vi "LVClass_HasoData Read HasoData - property.vi"(8 "error in (no error)":errorcluster, 11 "HasoData in":refnum<class "HasoData.lvclass">) -> (0 "error out":errorcluster, 2 "HasoData":T1, 3 "HasoData out":refnum<class "HasoData.lvclass">)   [LabVIEW 2020, in "HasoData.lvclass"]
uses:
  HasoData.lvclass
  Controls/ClassID.ctl
  HasoData.lvclass/HasoData.ctl
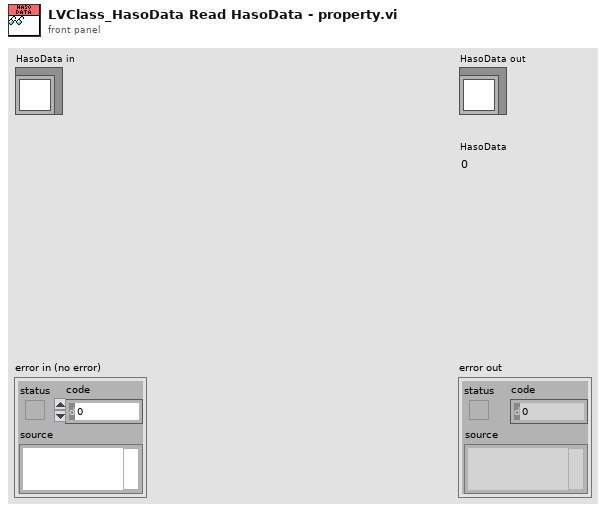
[diagram p1: front panel]
types:
  T1 = typedef "ClassID.ctl" = i64
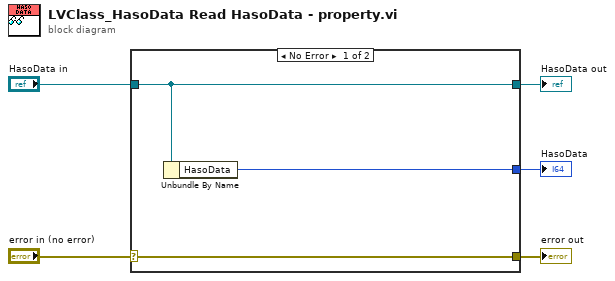
[diagram p0: block diagram]
diagram:
  n1 = case shown="No Error" "error in (no error)" {
    selector: "error in (no error)" -> [w8 w9]
    tunnel: [w8 w9] -> w4
    tunnel: [w7 w10] -> w2
    tunnel: "HasoData in" -> [w7 w10]
    tunnel: [w6 _] -> w1
    frame No Error {
      n2 = Unbundle By Name(w7) -> ("HasoData"=w6:T1)
    }
    frame Error {
    }
  }
  "error out" <- w4
  "HasoData out" <- w2
  "HasoData" <- w1
